vi "5.10 Main Demo.vi"() -> ()   [LabVIEW 2010]
uses:
  4-High Neurons/4.0-Timing Badass.ctl
  6-OCU Neurons/6.10 Occipital Neurons/6.10.1 LineDef.ctl
panel:
  out "Line Def":T1
  in  "Gains and Parameters":T2={"Control Gain"=0.0, "Line Def"=5.0, "Line Setpoint in Pixels"=0.0, "Low Pass Gain"=0.2, "Image Low Pass Gain"=0.2}
  out "Output to Mini Gauss":T3(plugin-control)
  out "Tiny Color Image":T3(plugin-control)
  in  "Input Fuzzy Blue Threshold":i32
  out "Super Heart Beat":T4
  out "Mini Gauss Control Signal":dbl[](array[numeric])
  in  "Pick the Movie":i32
  in  "Resample Scaling":i32=20 min=1 max=2000
  out "Disp Out":T3(plugin-control)
  in  "stop":bool
  in  "How Many Images":i32=300
  out "Main Display":T3(plugin-control)
  out "Picture location":path
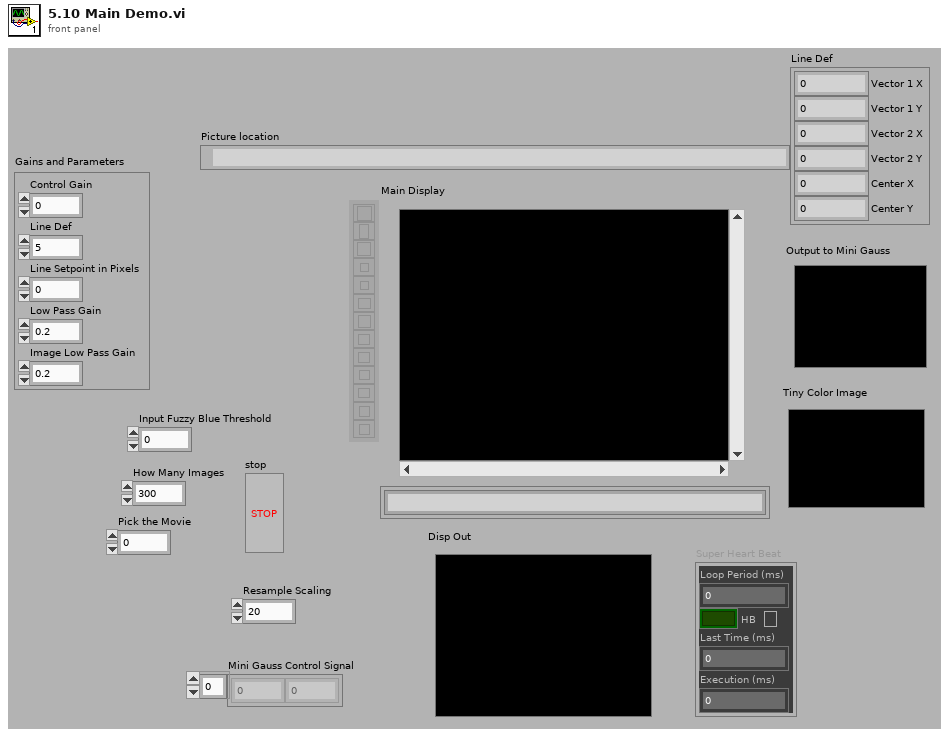
[diagram p1: front panel]
types:
  T1 = typedef "6.10.1 LineDef.ctl" = cluster{"Vector 1 X":dbl, "Vector 1 Y":dbl, "Vector 2 X":dbl, "Vector 2 Y":dbl, "Center X":dbl, "Center Y":dbl}
  T2 = cluster{"Control Gain":dbl, "Line Def":dbl, "Line Setpoint in Pixels":dbl, "Low Pass Gain":dbl, "Image Low Pass Gain":dbl}
  T3 = typedef "IMAQ Image.ctl" = refnum<image>
  T4 = typedef "4.0-Timing Badass.ctl" = cluster{"Loop Period (ms)":u32, "HB":bool, "Last Time (ms)":u32, "Execution (ms)":u32}
  T5 = typedef "5.10 Buffers Cluster.ctl" = cluster{"IMAQ Session":T6, "Buffer 0: Raw":T3, "Buffer 1: Resample":T3, "Buffer 2: Plane Extraction":T3, "Buffer 3: Re-mapping":T3, "Buffer 4: Overlay B/W":T3, "Buffer 5: Overlay Color":T3, "Buffer 6: Mask":T3, "Buffer 7: Masked Resample":T3}
  T6 = typedef "IMAQdx.ctl" = refnum<k21>
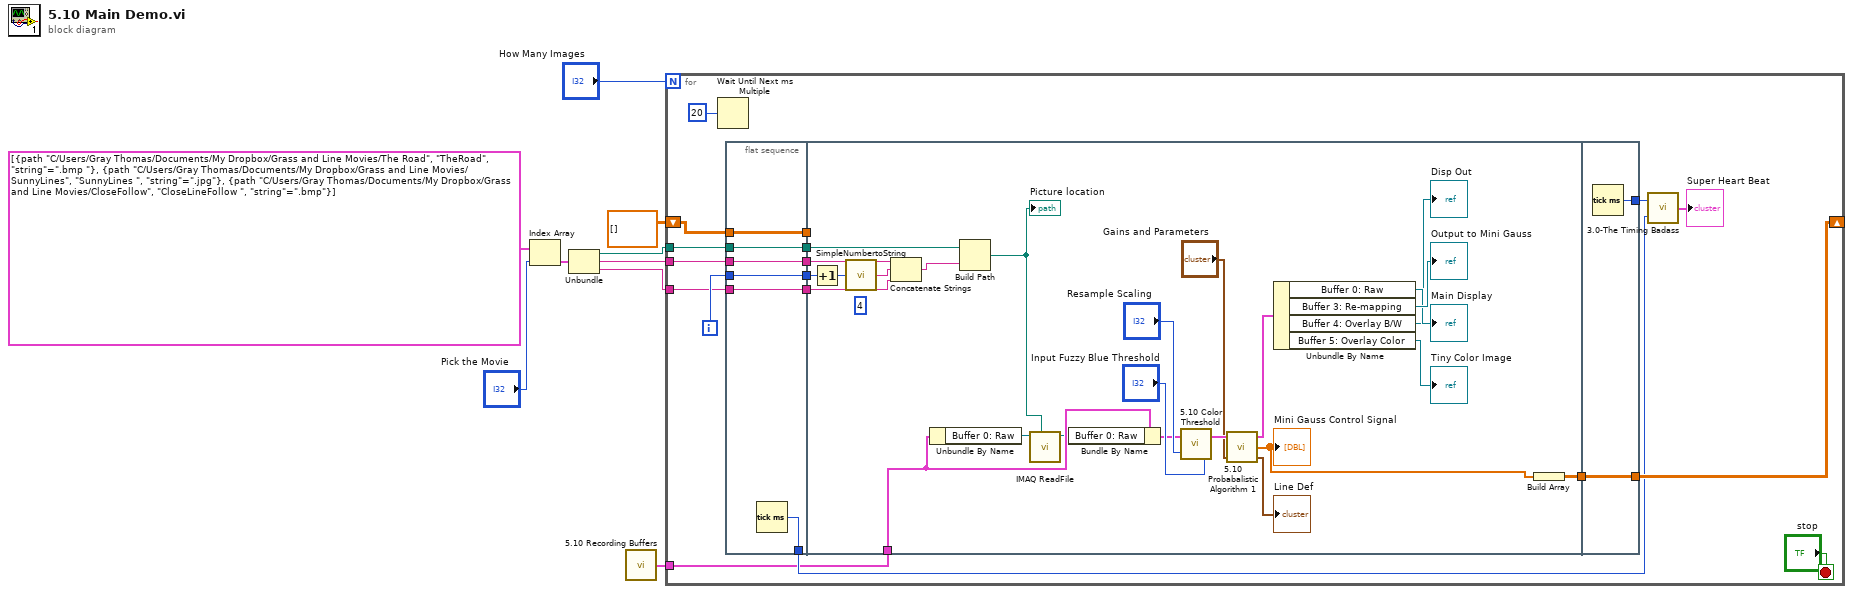
[diagram p0: block diagram]
diagram:
  n1 = Index Array(array=cluster{path, string, "string":string}[] [{path "C:/Users/Gray Thomas/Documents/My Dropbox/Grass and Line Movies/The Road", "TheRoad", "string"=".bmp "}, {path "C:/Users/Gray Thomas/Documents/My Dropbox/Grass and Line Movies/SunnyLines", "SunnyLines ", "string"=".jpg"}, {path "C:/Users/Gray Thomas/Documents/My Dropbox/Grass and Line Movies/CloseFollow", "CloseLineFollow ", "string"=".bmp"}], index="Pick the Movie") -> (element=w6:cluster{path, string, "string":string})
  n2 = Unbundle(w6) -> (w5:path, w4:string, "string"=w3:string)
  n3 = call "5.10 Recording Buffers.vi"() -> ("Recording Buffers"=w1:T5)  [unwired: 1 in]
  n4 = for {
    N: "How Many Images" -> [_]
    tunnel: w5 -> [w26]
    tunnel: w4 -> [w23]
    tunnel: w3 -> [w22]
    shift-right: [w21] -> _
    shift-left: dbl[][] [] ("Control Signal") -> [w20]
    tunnel: w1 -> [w10]
    i -> [w27]
    stop <- "stop" stop-if-true
    n5 = Wait Until Next ms Multiple(millisecond multiple=u32 20) -> ()  [unwired: 1 out]
    n6 = flat-sequence {
      tunnel: w20 -> [w29]
      tunnel: w22 -> [w30]
      tunnel: w23 -> [w31]
      tunnel: w26 -> [w32]
      tunnel: w27 -> [w33]
      tunnel: [w33] -> w18
      tunnel: [w32] -> w17
      tunnel: [w31] -> w16
      tunnel: [w30] -> w15
      tunnel: [w29] -> w14
      tunnel: [w28] -> w12
      tunnel: [w48] -> w19
      tunnel: w18 -> [w57]
      tunnel: w17 -> [w56]
      tunnel: w16 -> [w51]
      tunnel: w15 -> [w50]
      tunnel: w14 -> [_]
      tunnel: w10 -> [w43]
      tunnel: [w59] -> w21
      tunnel: w19 -> [w59]
      tunnel: [w58] -> w13
      frame #0 {
        n7 = Tick Count (ms)() -> (millisecond timer value=w28:u32)
      }
      frame #1 {
        (unwired) u32 4 ("Width")
        n8 = Increment(x=w57) -> (x+1=w52:i32)
        n9 = call "SimpleNumbertoString.vi"("Numeric"=w52) -> ("String"=w53:string)
        n10 = Concatenate Strings(w51, w53, w50) -> (w55:string)
        n11 = Unbundle By Name(w43) -> ("Buffer 0: Raw"=w42:T3)
        n12 = Build Path(base path=w56, name or relative path=w55) -> (appended path=w54:path)
        "Picture location" <- w54
        n13 = call "IMAQ ReadFile"("File Path"=w54, "Image"=w42) -> ("Image Out"=w41:T3)  [unwired: 5 in, 4 out]
        n14 = Bundle By Name(cluster=w43, "Buffer 0: Raw"=w41) -> (w44:T5)
        n15 = call "5.10 Color Threshold.vi"("Input Fuzzy Blue Threshold"="Input Fuzzy Blue Threshold", "Resample Scaling"="Resample Scaling", "Buffers In"=w44) -> ("Buffers Out"=w45:T5)
        n16 = call "5.10 Probabalistic Algorithm 1.vi"("Gains and Parameters"="Gains and Parameters", "Buffers Cluster In"=w45) -> ("Line Def"=→"Line Def":T1, "Control Signal"=w49:dbl[], "Buffers Cluster Out"=w40:T5)  [unwired: 1 in]
        "Mini Gauss Control Signal" <- w49
        n17 = Unbundle By Name(w40) -> ("Buffer 0: Raw"=→"Main Display":T3, "Buffer 3: Re-mapping"=→"Output to Mini Gauss":T3, "Buffer 4: Overlay B/W"=→"Disp Out":T3, "Buffer 5: Overlay Color"=→"Tiny Color Image":T3)
        n18 = Build Array(w49) -> (w48:dbl[][])
      }
      frame #2 {
        n19 = Tick Count (ms)() -> (millisecond timer value=w58:u32)
      }
    }
    n20 = call "3.0-The Timing Badass.vi"("Start"=w12, "End"=w13) -> ("Super Heart Beat"=→"Super Heart Beat":T4)
  }
